vi "Converter.vi"   [LabVIEW 2021]
doc: "Polymorphic VI to convert the target spec data to I2C data and I2C data to target spec data"
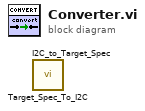
[diagram p0: block diagram]
diagram:
  n1 = call "Target_Spec_To_I2C.vi"() -> ()  [unwired: 15 in, 1 out]
  n2 = call "I2C_to_Target_Spec.vi"() -> ()  [unwired: 15 in, 1 out]
